vi "Import_Excel.vi"(10 "file path (dialog if empty)":path=path "C:/Users/DRX/Documents/Keysight/BenchVue/Test Flow/Exports/Flow 0.csv") -> (2 "voltagem":dbl[](array[numeric]))   [LabVIEW 2021]
uses:
  <vilib>/Utility/file.llb/Read Delimited Spreadsheet (DBL).vi
panel:
  out "error out":errorcluster
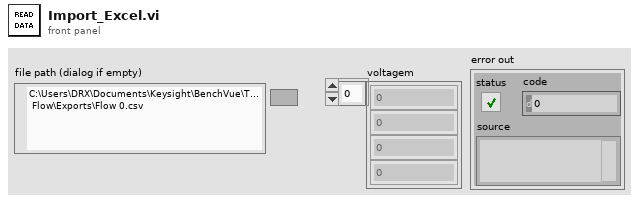
[diagram p1: front panel]
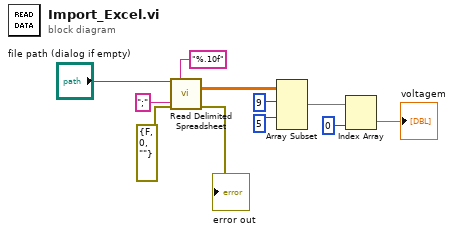
[diagram p0: block diagram]
diagram:
  n1 = call-poly <vilib>:"Read Delimited Spreadsheet.vi"("file path (dialog if empty)"="file path (dialog if empty)", "format (%.3f)"="%.10f", "error in (no error)"=errorcluster {"status"=FALSE, "code"=0, "source"=""}, "delimiter (\\t)"=";" ("delimiter (\\t)")) -> ("all rows"=w10:dbl[][], "error out"=→"error out":errorcluster)  [unwired: 6 in, 4 out]
  n2 = Array Subset(array=w10, index (row)=9 ("index"), index (col)=5 ("index")) -> (w7:dbl[][])  [unwired: 2 in]
  n3 = Index Array(array=w7, index (col)=0 ("disabled index (col)")) -> (element=→"voltagem":dbl[])  [unwired: 1 in]
